vi "final_VI.vi"() -> ()   [LabVIEW 2017]
uses:
  <vilib>/Analysis/baseanly.llb/Mean (DBL).vi
  <instrlib>/Lake Shore Cryotronics 332/Lake Shore Cryotronics 332.lvlib
  <instrlib>/Keithley 6517/Keithley 6517.lvlib
  <vilib>/Analysis/NI_AALBase.lvlib
panel:
  out "DURING COOLING":cluster{dbl[], dbl[]}(graph)
  in  "milliseconds to wait 2":u32
  in  "area 2":dbl
  in  "length 2":dbl
  out "x/y 2":dbl
  in  "V-source Amplitude \n 2":dbl format="%.6e"
  in  "Number of readings of Voltage 2":dbl
  in  "Visa resource Manager for keithley 2":refnum<visa-resource-name>
  out "DURING HEATING":cluster{dbl[], dbl[]}(graph)
  in  "milliseconds to wait":u32
  in  "area":dbl
  in  "length":dbl
  out "x/y":dbl
  in  "V-source Amplitude":dbl format="%.6e"
  in  "Number of readings of Voltage":dbl
  in  "Visa resource Manager for keithley":refnum<visa-resource-name>
  in  "Rate(D)":dbl min=0.0 max=200.0 step=1.0
  in  "Reset (I) (0.0)":dbl min=0.0 max=1000.0 step=0.1 format="%.1f"
  in  "Gain (P)":dbl min=0.0 max=1000.0 step=0.1 format="%.1f"
  in  "Manual Output":dbl min=0.0 max=100.0 step=0.001 format="%.3f"
  in  "Heater Range ()":u16(ring) items=["Off", "Low (0.5W)", "Med (5W)", "High (50W)"]
  in  "Enable Powerup ()":bool
  in  "Control Mode":u16(ring) items=["Manual PID", "Zone", "Open Loop", "AutoTune PID", "AutoTune PI", "AutoTune P"]
  out "return count":u32
  out "?":u32
  out "error out 2":errorcluster
  in  "error in (no error)":errorcluster
  out "error out":errorcluster
  out "return count 2":u32
  out "?":u32
  in  "error in (no error) 2":errorcluster
  out "error out 3":errorcluster
  in  "Visa resource Manager for lakeshore":refnum<visa-resource-name>
  in  "time interval to wait":dbl
  in  "Temo diff":dbl
  in  "End Temp":dbl
  in  "Start Temp":dbl
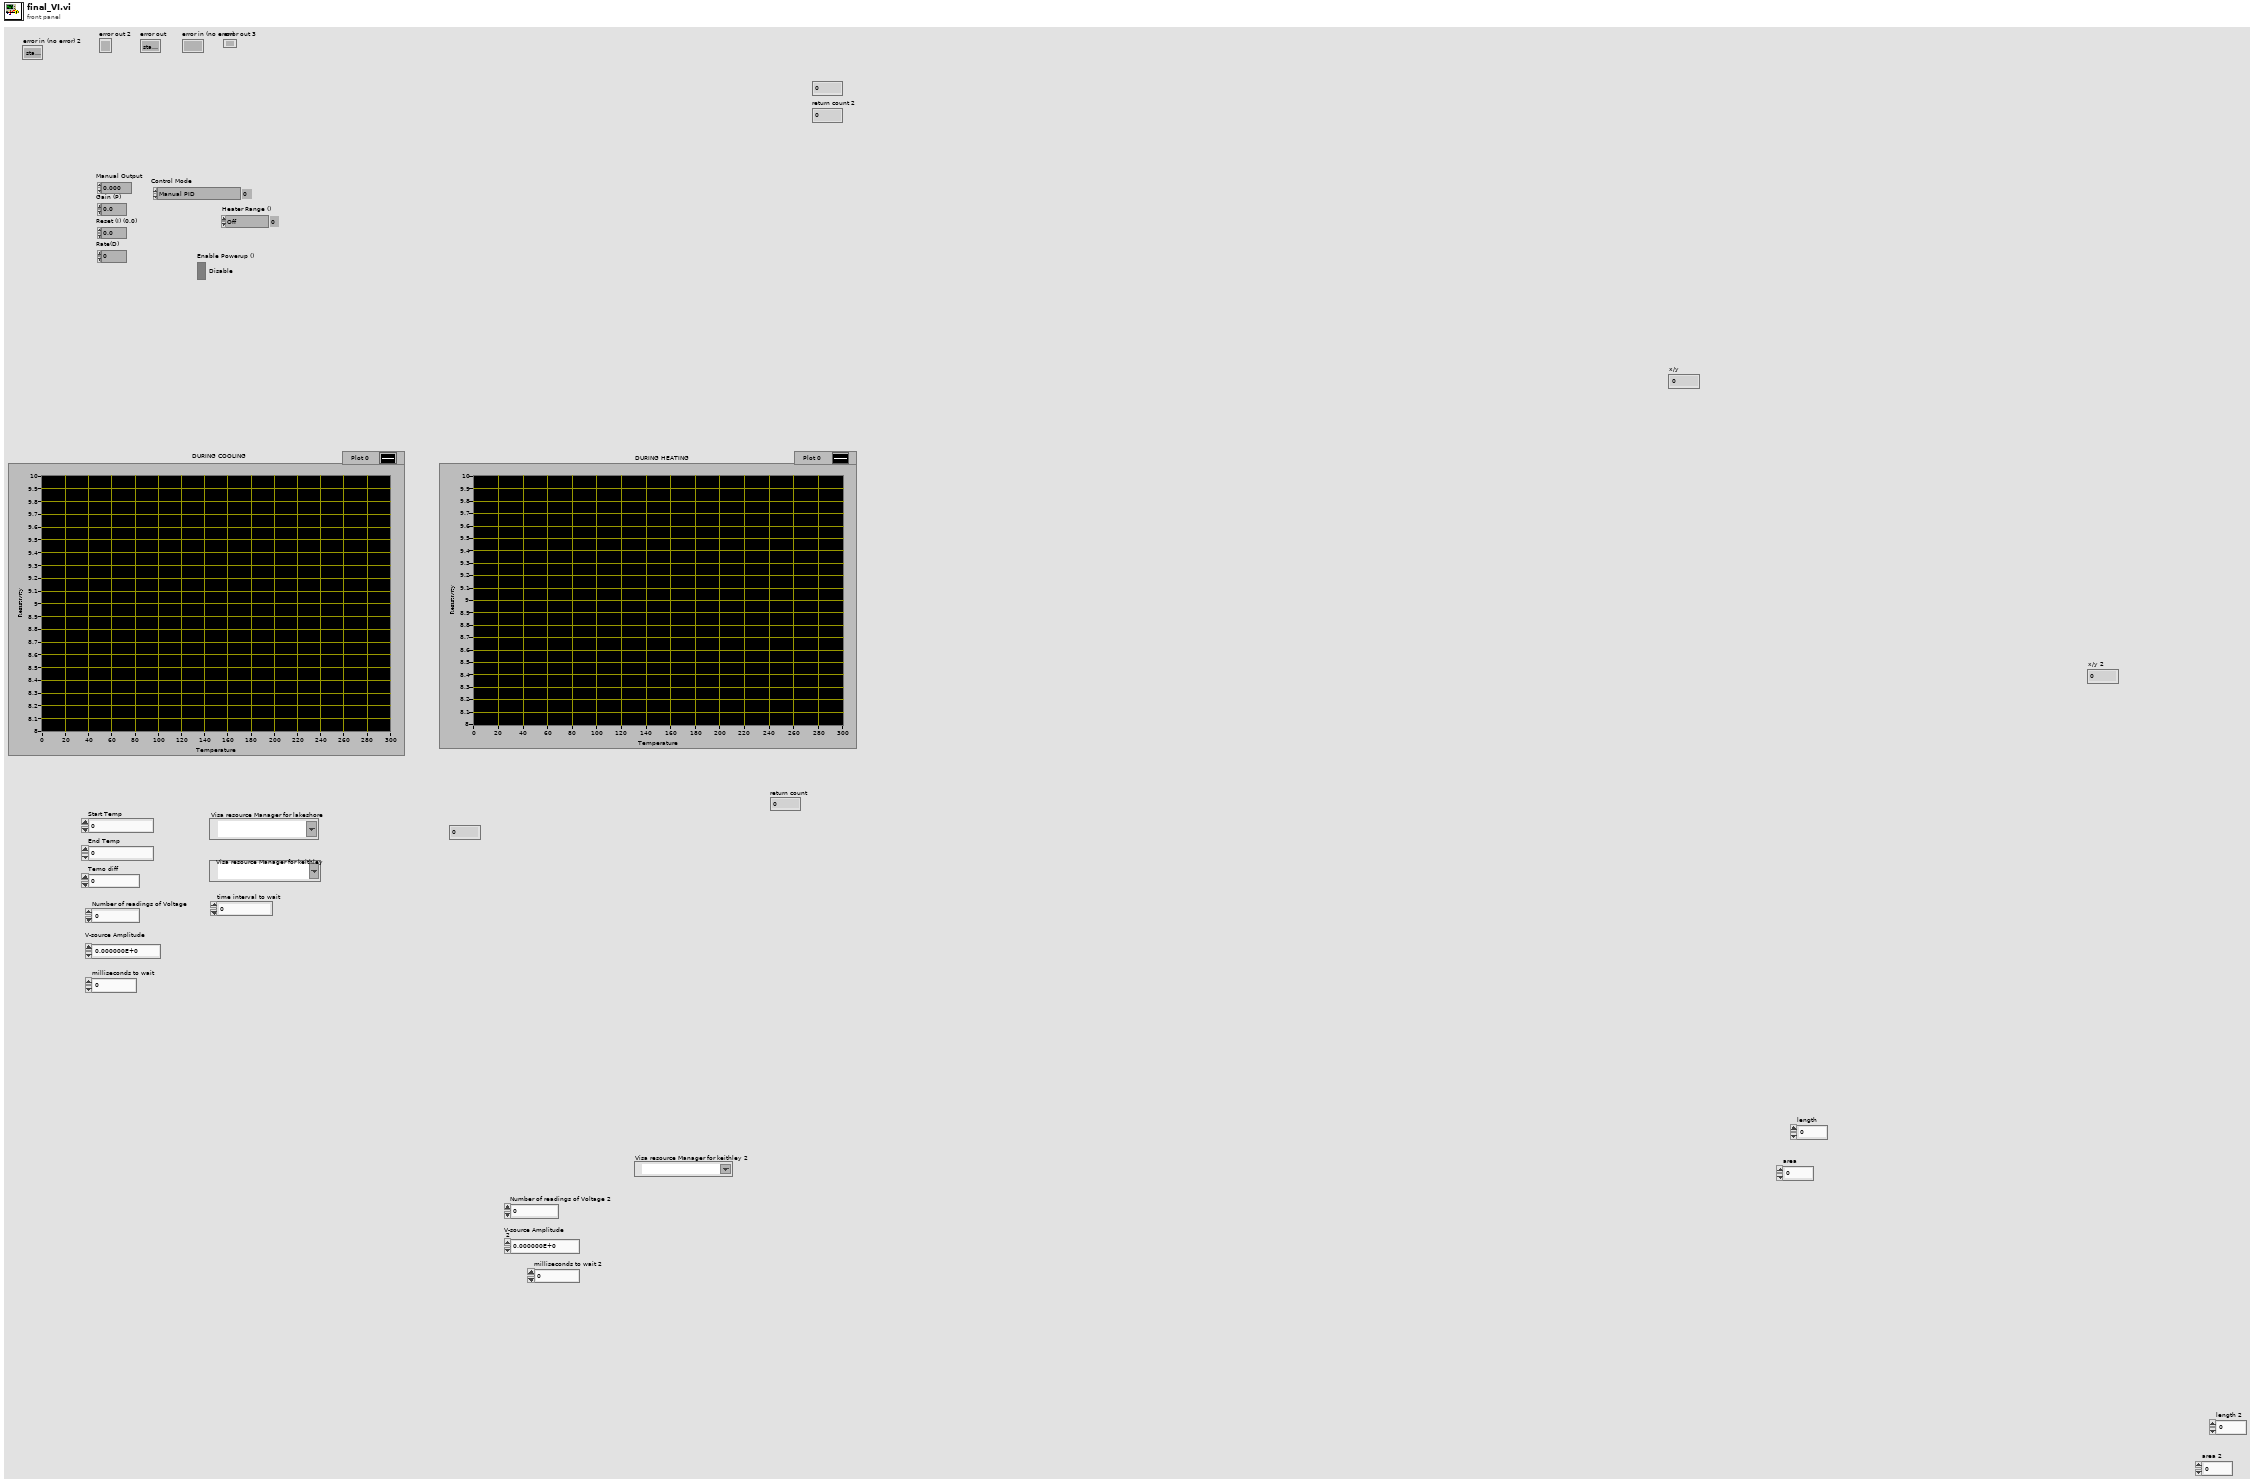
[diagram p1: front panel]
types:
  T1 = cluster{"Measurement":dbl, "Units":string, "Time Stamp and Date":string, "Reading #":dbl, "Channel #":dbl}
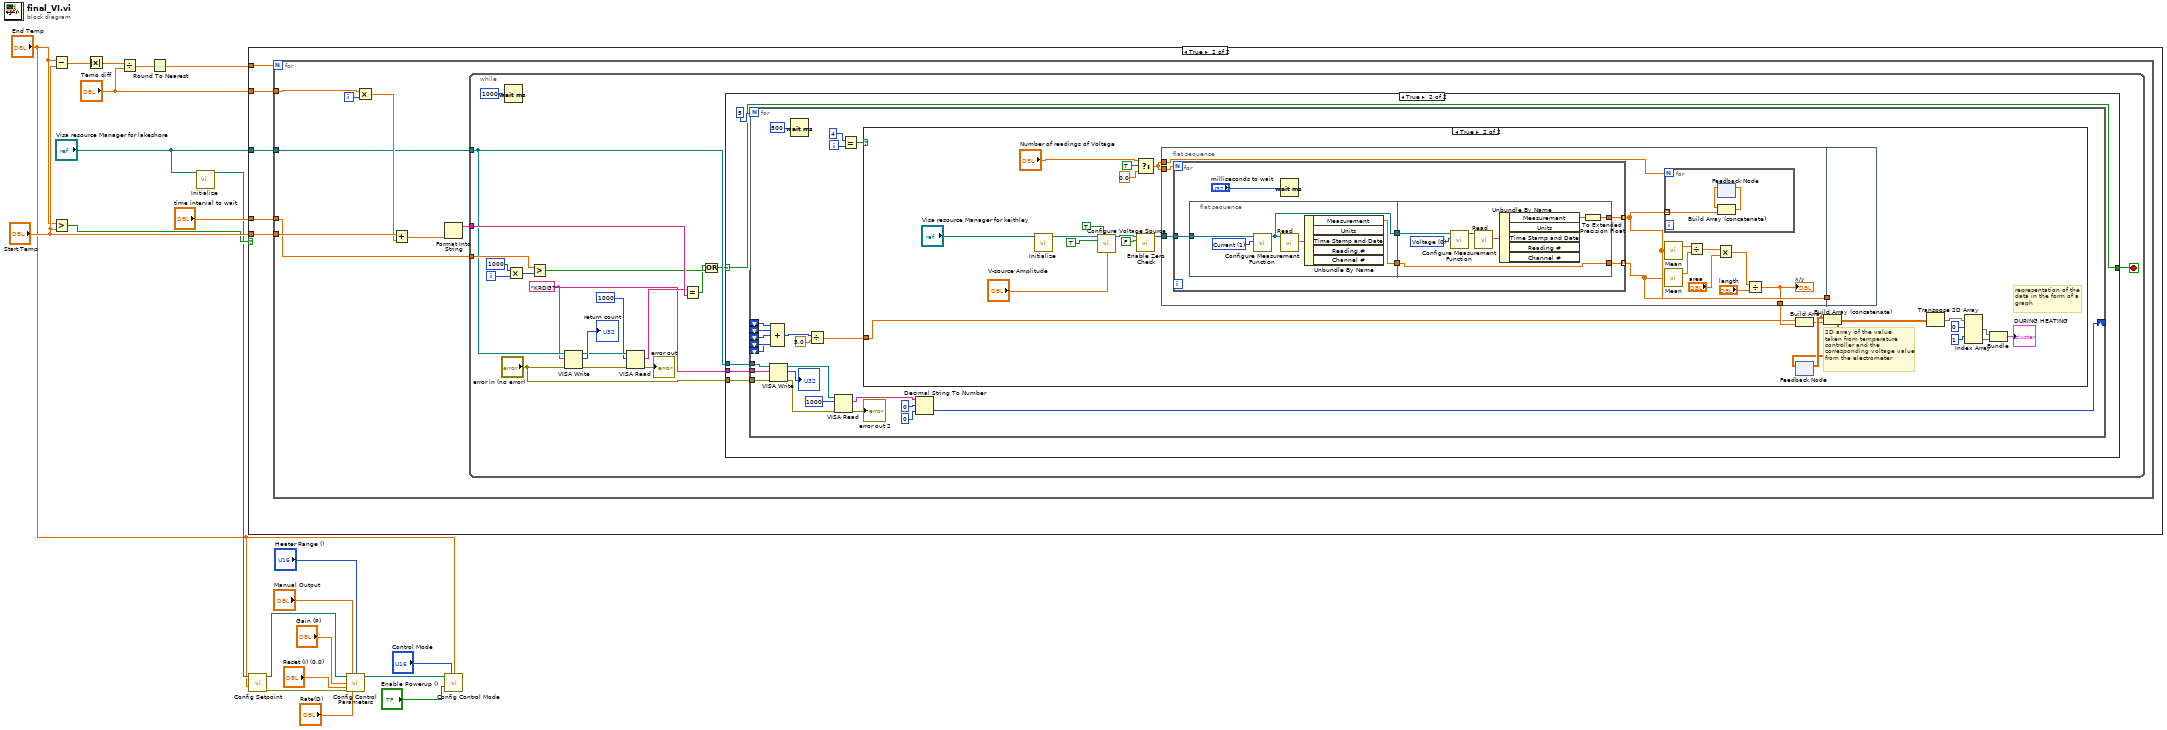
[diagram p0: block diagram]
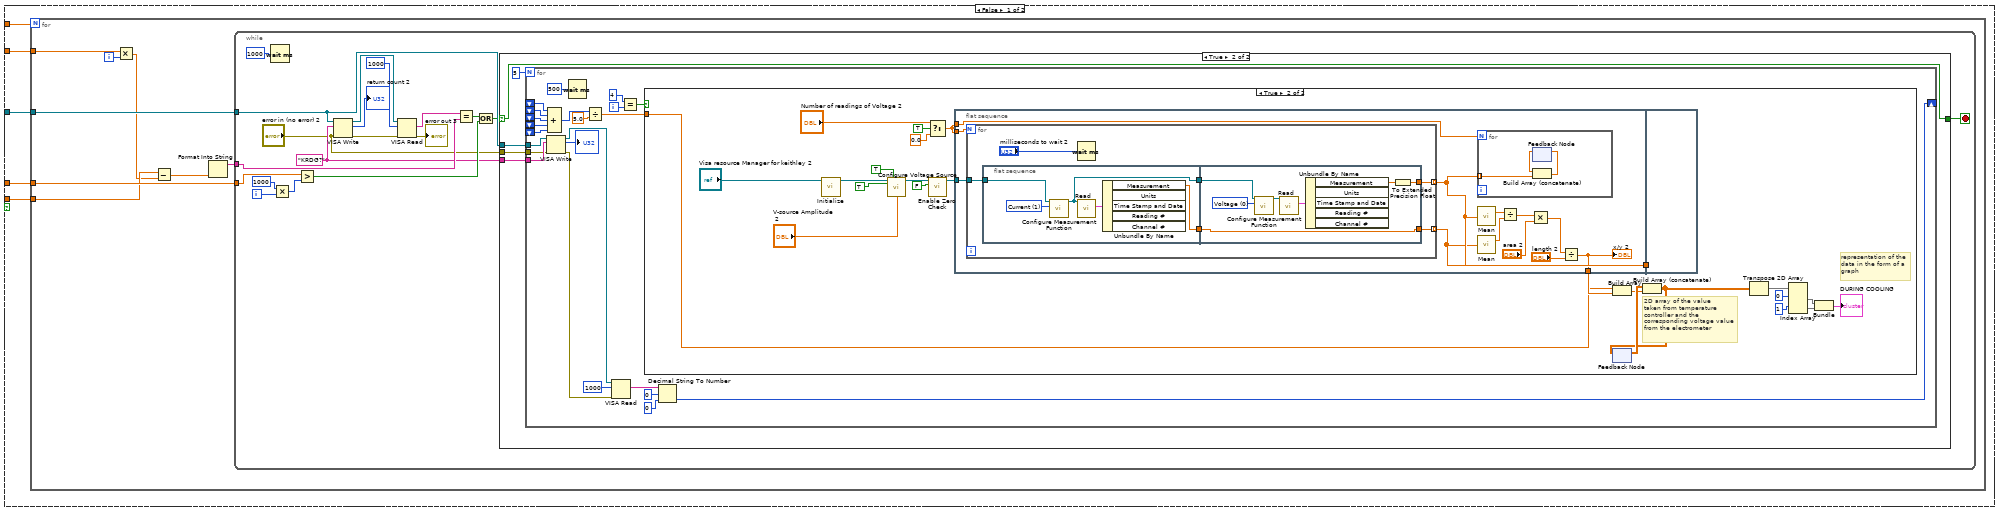
[diagram p2: hidden frame]
diagram:
  n1 = Subtract(x="End Temp", y="Start Temp") -> (x-y=w15:dbl)
  n2 = Greater?(x="End Temp", y="Start Temp") -> (0:w16:bool)
  n3 = Absolute Value(x=w15) -> (abs(x)=w14:dbl)
  n4 = Divide(x=w14, y="Temo diff") -> (x/y=w21:dbl)
  n5 = Round To Nearest(number=w21) -> (nearest integer value=w20:dbl)
  n6 = call <instrlib>:"Initialize.vi"("VISA resource name"="Visa resource Manager for lakeshore") -> ("VISA resource name out"=w13:refnum<visa-resource-name>)  [unwired: 13 in, 1 out]
  n7 = case shown="True" w16 {
    tunnel: w20 -> [w25 w145]
    tunnel: "Temo diff" -> [w22 w144]
    tunnel: "Start Temp" -> [w23 w143]
    tunnel: "Visa resource Manager for lakeshore" -> [w26 w142]
    tunnel: "time interval to wait" -> [w24 w141]
    frame False {
      n8 = for {
        N: w25 -> [_]
        tunnel: w22 -> [w34]
        tunnel: w23 -> [w29]
        tunnel: w26 -> [w33]
        tunnel: w24 -> [w32]
        i -> [w31]
        n9 = Multiply(x=w34, y=w31) -> (x*y=w28:dbl)
        n10 = Subtract(x=w29, y=w28) -> (x-y=w27:dbl)
        n11 = Format Into String(w27) -> (resulting string=w30:string)  [unwired: 3 in, 1 out]
        n12 = while {
          tunnel: w33 -> [w42]
          tunnel: w30 -> [w48]
          tunnel: w32 -> [w43]
          i -> [w46]
          stop <- w37 stop-if-true
          w40 = "KRDG?" ("write buffer")
          n13 = Wait (ms)(milliseconds to wait=u32 1000) -> ()  [unwired: 1 out]
          n14 = Multiply(x=1000, y=w46) -> (x*y=w44:i32)
          n15 = Greater?(x=w43, y=w44) -> (0:w41:bool)
          n16 = VISA Write(VISA resource name=w42, write buffer=w40, error in (no error)="error in (no error) 2") -> (VISA resource name out=w52:refnum<visa-resource-name>, return count=→"return count 2":u32, error out=w50:errorcluster)
          n17 = VISA Read(VISA resource name=w52, byte count=u32 1000, error in (no error)=w50) -> (read buffer=w47:string, error out=→"error out 3":errorcluster)  [unwired: 2 out]
          n18 = Equal?(x=w47, y=w48) -> (x = y?=w39:bool)
          n19 = Or(x=w39, y=w41) -> (x .or. y?=w38:bool)
          n20 = case shown="True" w38 {
            selector: w38 -> [w54 w56]
            tunnel: w42 -> [_ w58]
            tunnel: w40 -> [_ w57]
            tunnel: [w54 w56] -> w37
            tunnel: "error in (no error) 2" -> [_ w55]
            frame False {
            }
            frame True {
              n21 = for {
                N: 5 -> [_]
                tunnel: w58 -> [w79]
                shift-right: [w73] -> _
                shift-left: _ -> [w72]
                shift-left: _ -> [w71]
                shift-left: _ -> [w70]
                shift-left: _ -> [w69]
                shift-left: _ -> [w68]
                tunnel: w57 -> [w63]
                tunnel: w55 -> [w60]
                i -> [w65]
                n22 = VISA Write(VISA resource name=w79, write buffer=w63, error in (no error)=w60) -> (VISA resource name out=w78:refnum<visa-resource-name>, return count=→"?":u32, error out=w81:errorcluster)
                n23 = Compound Arithmetic op=ADD(w72, w71, w70, w69, w68) -> (w66:i32)
                n24 = Wait (ms)(milliseconds to wait=u32 500) -> ()  [unwired: 1 out]
                n25 = Divide(x=w66, y=5.0) -> (x/y=w62:dbl)
                n26 = VISA Read(VISA resource name=w78, byte count=u32 1000, error in (no error)=w81) -> (read buffer=w76:string)  [unwired: 3 out]
                n27 = Equal?(x=4, y=w65) -> (x = y?=w61:bool)
                n28 = case shown="True" w61 {
                  tunnel: w62 -> [_ w83]
                  frame False {
                  }
                  frame True {
                    # "representation of the \ndata in the form of a\ngraph"
                    # "2D array of the value\ntaken from temperature\ncontroller and the\ncorresponding voltage value \nfrom the electrometer"
                    n29 = call <instrlib>:"Initialize.vi"("VISA resource name"="Visa resource Manager for keithley 2") -> ("VISA resource name out"=w101:refnum<visa-resource-name>)  [unwired: 9 in, 1 out]
                    n30 = call <instrlib>:"Configure Voltage Source.vi"("VISA resource name"=w101, "Enable LO Connection (F: Disable)"=TRUE, "Enable V-source (F: Disable)"=TRUE, "V-source Amplitude (0.000000E+0)"="V-source Amplitude \n 2") -> ("VISA resource name out"=w100:refnum<visa-resource-name>)  [unwired: 10 in, 1 out]
                    n31 = Select(t="Number of readings of Voltage 2", s=TRUE, f=0.0) -> (s? t:f=w103:dbl)
                    n32 = call <instrlib>:"Enable Zero Check.vi"("Enable Zero Check (T: Enable)"=FALSE, "VISA resource name"=w100) -> ("VISA resource name out"=w96:refnum<visa-resource-name>)  [unwired: 8 in, 1 out]
                    n33 = flat-sequence {
                      tunnel: w96 -> [w119]
                      tunnel: w103 -> [w118]
                      tunnel: [w113] -> w107
                      tunnel: [w115] -> w106
                      tunnel: w103 -> [w114]
                      tunnel: [w108] -> w84
                      tunnel: w107 -> [_]
                      tunnel: w106 -> [_]
                      frame #0 {
                        n34 = for {
                          N: w118 -> [_]
                          tunnel: w119 -> [w126]
                          tunnel: [w127] -> w113 mode=indexing
                          tunnel: [w123] -> w115 mode=indexing
                          n35 = flat-sequence {
                            tunnel: w126 -> [w131]
                            tunnel: [w132] -> w125
                            tunnel: [w130] -> w124
                            tunnel: [w140] -> w127
                            tunnel: w125 -> [w140]
                            tunnel: w124 -> [w137]
                            tunnel: [w134] -> w123
                            frame #0 {
                              w129 = 1 items=["Voltage", "Current", "Resistance", "Charge"] ("Measurement Function (0: Voltage)")
                              n36 = call <instrlib>:"Configure Measurement Function.vi"("Measurement Function (0: Voltage)"=w129, "VISA resource name"=w131) -> ("VISA resource name out"=w130:refnum<visa-resource-name>)  [unwired: 8 in, 1 out]
                              n37 = call <instrlib>:"Read.vi"("VISA resource name"=w130) -> ("Measurement"=w133:T1)  [unwired: 8 in, 2 out]
                              n38 = Unbundle By Name(w133) -> ("Measurement"=w132:dbl)  [unwired: 4 out]
                            }
                            frame #1 {
                              w136 = 0 items=["Voltage", "Current", "Resistance", "Charge"] ("Measurement Function (0: Voltage)")
                              n39 = call <instrlib>:"Configure Measurement Function.vi"("Measurement Function (0: Voltage)"=w136, "VISA resource name"=w137) -> ("VISA resource name out"=w138:refnum<visa-resource-name>)  [unwired: 8 in, 1 out]
                              n40 = call <instrlib>:"Read.vi"("VISA resource name"=w138) -> ("Measurement"=w139:T1)  [unwired: 8 in, 2 out]
                              n41 = Unbundle By Name(w139) -> ("Measurement"=w135:dbl)  [unwired: 4 out]
                              n42 = To Extended Precision Float(1:w135) -> (0:w134:ext)
                            }
                          }
                          n43 = Wait (ms)(milliseconds to wait="milliseconds to wait 2") -> ()  [unwired: 1 out]
                        }
                        n44 = for {
                          N: w114 -> [_]
                          tunnel: w115 -> [w122] mode=indexing
                          n45 = feedback #1() -> (w121:ext[])  [unwired: 1 in]
                          n46 = Build Array (concatenate)(w121, w122) -> (w120:ext[])
                          n47 = feedback-in #1(w120) -> ()
                        }
                        n48 = call-poly <vilib>:"Mean.vi"("X"=w115) -> ("mean"=w116:dbl)  [unwired: 1 out]
                        n49 = call-poly <vilib>:"Mean.vi"("X"=w113) -> ("mean"=w117:dbl)  [unwired: 1 out]
                        n50 = Divide(x=w116, y=w117) -> (x/y=w111:dbl)
                        n51 = Multiply(x=w111, y="area 2") -> (x*y=w109:dbl)
                        n52 = Divide(x=w109, y="length 2") -> (x/y=w108:dbl)
                        "x/y 2" <- w108
                      }
                      frame #1 {
                      }
                    }
                    n53 = Build Array(w83, w84) -> (w85:dbl[])
                    n54 = feedback #2() -> (w93:dbl[][])  [unwired: 1 in]
                    n55 = Build Array (concatenate)(w93, w85) -> (w86:dbl[][])
                    n56 = feedback-in #2(w86) -> ()
                    n57 = Transpose 2D Array(2D array=w86) -> (transposed array=w87:dbl[][])
                    n58 = Index Array(array=w87, index (row) #1=0 ("index (row)"), index (row) #2=1 ("index (row)")) -> (element #1=w90:dbl[], element #2=w89:dbl[])  [unwired: 2 in]
                    n59 = Bundle(w90, w89) -> (→"DURING COOLING":cluster{dbl[], dbl[]})  [unwired: 1 in]
                  }
                }
                n60 = Decimal String To Number(string=w76, offset=0, default (0L)=0 ("default (0 I32)")) -> (number=w73:i32)  [unwired: 1 out]
              }
            }
          }
        }
      }
    }
    frame True {
      n61 = for {
        N: w145 -> [_]
        tunnel: w144 -> [w153]
        tunnel: w143 -> [w152]
        tunnel: w142 -> [w149]
        tunnel: w141 -> [w148]
        i -> [w147]
        n62 = Multiply(x=w153, y=w147) -> (x*y=w151:dbl)
        n63 = Add(x=w152, y=w151) -> (x+y=w150:dbl)
        n64 = Format Into String(w150) -> (resulting string=w146:string)  [unwired: 3 in, 1 out]
        n65 = while {
          tunnel: w149 -> [w161]
          tunnel: w146 -> [w167]
          tunnel: w148 -> [w162]
          i -> [w165]
          stop <- w156 stop-if-true
          w159 = "KRDG?" ("write buffer")
          n66 = Wait (ms)(milliseconds to wait=u32 1000) -> ()  [unwired: 1 out]
          n67 = Multiply(x=1000, y=w165) -> (x*y=w163:i32)
          n68 = Greater?(x=w162, y=w163) -> (0:w160:bool)
          n69 = VISA Write(VISA resource name=w161, write buffer=w159, error in (no error)="error in (no error)") -> (VISA resource name out=w171:refnum<visa-resource-name>, return count=→"return count":u32, error out=w169:errorcluster)
          n70 = VISA Read(VISA resource name=w171, byte count=u32 1000, error in (no error)=w169) -> (read buffer=w166:string, error out=→"error out":errorcluster)  [unwired: 2 out]
          n71 = Equal?(x=w166, y=w167) -> (x = y?=w158:bool)
          n72 = Or(x=w158, y=w160) -> (x .or. y?=w157:bool)
          n73 = case shown="True" w157 {
            selector: w157 -> [w173 w175]
            tunnel: w161 -> [_ w177]
            tunnel: w159 -> [_ w176]
            tunnel: [w173 w175] -> w156
            tunnel: "error in (no error)" -> [_ w174]
            frame False {
            }
            frame True {
              n74 = for {
                N: 5 -> [_]
                tunnel: w177 -> [w199]
                shift-right: [w193] -> _
                shift-left: _ -> [w192]
                shift-left: _ -> [w191]
                shift-left: _ -> [w190]
                shift-left: _ -> [w189]
                shift-left: _ -> [w188]
                tunnel: w176 -> [w183]
                tunnel: w174 -> [w181]
                i -> [w185]
                n75 = VISA Write(VISA resource name=w199, write buffer=w183, error in (no error)=w181) -> (VISA resource name out=w198:refnum<visa-resource-name>, return count=→"?":u32, error out=w201:errorcluster)
                n76 = Compound Arithmetic op=ADD(w192, w191, w190, w189, w188) -> (w186:i32)
                n77 = Wait (ms)(milliseconds to wait=u32 500) -> ()  [unwired: 1 out]
                n78 = Divide(x=w186, y=5.0) -> (x/y=w182:dbl)
                n79 = VISA Read(VISA resource name=w198, byte count=u32 1000, error in (no error)=w201) -> (read buffer=w196:string, error out=→"error out 2":errorcluster)  [unwired: 2 out]
                n80 = Equal?(x=4, y=w185) -> (x = y?=w179:bool)
                n81 = case shown="True" w179 {
                  tunnel: w182 -> [_ w203]
                  frame False {
                  }
                  frame True {
                    # "representation of the \ndata in the form of a\ngraph"
                    # "2D array of the value\ntaken from temperature\ncontroller and the\ncorresponding voltage value \nfrom the electrometer"
                    n82 = call <instrlib>:"Initialize.vi"("VISA resource name"="Visa resource Manager for keithley") -> ("VISA resource name out"=w221:refnum<visa-resource-name>)  [unwired: 9 in, 1 out]
                    n83 = call <instrlib>:"Configure Voltage Source.vi"("VISA resource name"=w221, "Enable LO Connection (F: Disable)"=TRUE, "Enable V-source (F: Disable)"=TRUE, "V-source Amplitude (0.000000E+0)"="V-source Amplitude") -> ("VISA resource name out"=w220:refnum<visa-resource-name>)  [unwired: 10 in, 1 out]
                    n84 = Select(t="Number of readings of Voltage", s=TRUE, f=0.0) -> (s? t:f=w223:dbl)
                    n85 = call <instrlib>:"Enable Zero Check.vi"("Enable Zero Check (T: Enable)"=FALSE, "VISA resource name"=w220) -> ("VISA resource name out"=w216:refnum<visa-resource-name>)  [unwired: 8 in, 1 out]
                    n86 = flat-sequence {
                      tunnel: w216 -> [w239]
                      tunnel: w223 -> [w238]
                      tunnel: [w233] -> w227
                      tunnel: [w235] -> w226
                      tunnel: w223 -> [w234]
                      tunnel: [w228] -> w204
                      tunnel: w227 -> [_]
                      tunnel: w226 -> [_]
                      frame #0 {
                        n87 = for {
                          N: w238 -> [_]
                          tunnel: w239 -> [w246]
                          tunnel: [w247] -> w233 mode=indexing
                          tunnel: [w243] -> w235 mode=indexing
                          n88 = flat-sequence {
                            tunnel: w246 -> [w251]
                            tunnel: [w252] -> w245
                            tunnel: [w250] -> w244
                            tunnel: [w260] -> w247
                            tunnel: w245 -> [w260]
                            tunnel: w244 -> [w257]
                            tunnel: [w254] -> w243
                            frame #0 {
                              w249 = 1 items=["Voltage", "Current", "Resistance", "Charge"] ("Measurement Function (0: Voltage)")
                              n89 = call <instrlib>:"Configure Measurement Function.vi"("Measurement Function (0: Voltage)"=w249, "VISA resource name"=w251) -> ("VISA resource name out"=w250:refnum<visa-resource-name>)  [unwired: 8 in, 1 out]
                              n90 = call <instrlib>:"Read.vi"("VISA resource name"=w250) -> ("Measurement"=w253:T1)  [unwired: 8 in, 2 out]
                              n91 = Unbundle By Name(w253) -> ("Measurement"=w252:dbl)  [unwired: 4 out]
                            }
                            frame #1 {
                              w256 = 0 items=["Voltage", "Current", "Resistance", "Charge"] ("Measurement Function (0: Voltage)")
                              n92 = call <instrlib>:"Configure Measurement Function.vi"("Measurement Function (0: Voltage)"=w256, "VISA resource name"=w257) -> ("VISA resource name out"=w258:refnum<visa-resource-name>)  [unwired: 8 in, 1 out]
                              n93 = call <instrlib>:"Read.vi"("VISA resource name"=w258) -> ("Measurement"=w259:T1)  [unwired: 8 in, 2 out]
                              n94 = Unbundle By Name(w259) -> ("Measurement"=w255:dbl)  [unwired: 4 out]
                              n95 = To Extended Precision Float(1:w255) -> (0:w254:ext)
                            }
                          }
                          n96 = Wait (ms)(milliseconds to wait="milliseconds to wait") -> ()  [unwired: 1 out]
                        }
                        n97 = for {
                          N: w234 -> [_]
                          tunnel: w235 -> [w242] mode=indexing
                          n98 = feedback #3() -> (w241:ext[])  [unwired: 1 in]
                          n99 = Build Array (concatenate)(w241, w242) -> (w240:ext[])
                          n100 = feedback-in #3(w240) -> ()
                        }
                        n101 = call-poly <vilib>:"Mean.vi"("X"=w235) -> ("mean"=w236:dbl)  [unwired: 1 out]
                        n102 = call-poly <vilib>:"Mean.vi"("X"=w233) -> ("mean"=w237:dbl)  [unwired: 1 out]
                        n103 = Divide(x=w236, y=w237) -> (x/y=w231:dbl)
                        n104 = Multiply(x=w231, y="area") -> (x*y=w229:dbl)
                        n105 = Divide(x=w229, y="length") -> (x/y=w228:dbl)
                        "x/y" <- w228
                      }
                      frame #1 {
                      }
                    }
                    n106 = Build Array(w203, w204) -> (w205:dbl[])
                    n107 = feedback #4() -> (w213:dbl[][])  [unwired: 1 in]
                    n108 = Build Array (concatenate)(w213, w205) -> (w206:dbl[][])
                    n109 = feedback-in #4(w206) -> ()
                    n110 = Transpose 2D Array(2D array=w206) -> (transposed array=w207:dbl[][])
                    n111 = Index Array(array=w207, index (row) #1=0 ("index (row)"), index (row) #2=1 ("index (row)")) -> (element #1=w210:dbl[], element #2=w209:dbl[])  [unwired: 2 in]
                    n112 = Bundle(w210, w209) -> (→"DURING HEATING":cluster{dbl[], dbl[]})  [unwired: 1 in]
                  }
                }
                n113 = Decimal String To Number(string=w196, offset=0, default (0L)=0 ("default (0 I32)")) -> (number=w193:i32)  [unwired: 1 out]
              }
            }
          }
        }
      }
    }
  }
  n114 = call <instrlib>:"Config Setpoint.vi"("Setpoint (0.0000)"="End Temp", "VISA resource name"=w13) -> ("error out"=w9:errorcluster, "VISA resource name out"=w10:refnum<visa-resource-name>)  [unwired: 8 in]
  n115 = call <instrlib>:"Config Control Parameters.vi"("VISA resource name"=w10, "Manual Output (0.000)"="Manual Output", "Heater Range (0: Off)"="Heater Range ()", "Gain (P) (0.0)"="Gain (P)", "Reset (I) (0.0)"="Reset (I) (0.0)", "error in (no error)"=w9, "Rate (D) (0)"="Rate(D)") -> ("VISA resource name out"=w8:refnum<visa-resource-name>)  [unwired: 7 in, 1 out]
  n116 = call <instrlib>:"Config Control Mode.vi"("VISA resource name"=w8, "Control Mode (0: Manual PID)"="Control Mode", "Setpoint Units (0: Kelvin)"="End Temp", "Enable Powerup (F: Enable)"="Enable Powerup ()") -> ()  [unwired: 10 in, 2 out]
